vi "ConvertVSEnumToPath.vi"(10 "Source.Path Type":T1(ring), 11 "Path In":path) -> (3 "appended path":path)   [LabVIEW 2015, in "Configuration Tool.lvlib"]
uses:
  Configuration Tool.lvlib
  <vilib>/Utility/sysdir.llb/System Directory Type.ctl
  Global Settings.vi
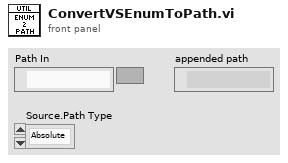
[diagram p1: front panel]
types:
  T1 = enum16{"Absolute", "To Base", "To Common Doc Dir", "To Application Data Dir"}
  T2 = typedef "System Directory Type.ctl" = i32
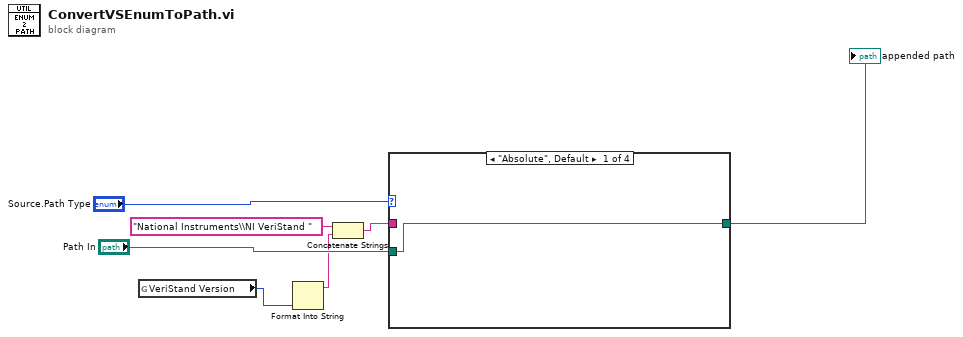
[diagram p0: block diagram]
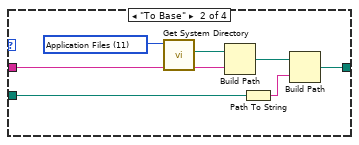
[diagram p2: hidden frame]
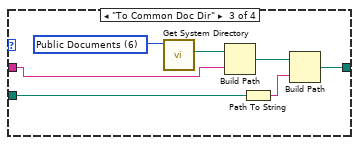
[diagram p3: hidden frame]
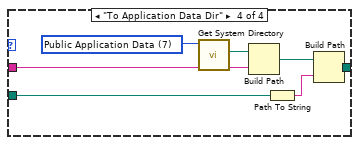
[diagram p4: hidden frame]
diagram:
  n1 = global read "Global Settings.vi" "VeriStand Version"() -> (w4:enum16{"2013", "2014", "2015", "2016"})
  n2 = Format Into String(w4) -> (resulting string=w2:string)  [unwired: 3 in, 1 out]
  n3 = Concatenate Strings("National Instruments\\NI VeriStand " ("name or relative path"), w2) -> (w1:string)
  n4 = case shown="\"Absolute\", Default" "Source.Path Type" {
    tunnel: "Path In" -> [w8 w11 w18 w25]
    tunnel: [w8 w10 w17 w24] -> w7
    tunnel: w1 -> [_ w9 w16 w23]
    frame "Absolute", Default {
    }
    frame "To Base" {
      w15 = T2 11 items=["User Home"=0, "User Desktop"=1, "User Documents"=2, "User Application Data"=3, "User Preferences"=4, "User Temporary"=5, "Public Documents"=6, "Public Application Data"=7, "Public Preferences"=8, "Public Cache"=13, "System Core Libraries"=9, "System Installed Libraries"=10, "Application Files"=11, "Boot Volume Root"=12] ("system directory type")
      n5 = call <vilib>:"Get System Directory.vi"("system directory type"=w15) -> ("system directory"=w14:path)  [unwired: 10 in]
      n6 = Build Path(base path=w14, name or relative path=w9) -> (appended path=w13:path)
      n7 = Path To String(path=w11) -> (string=w12:string)
      n8 = Build Path(base path=w13, name or relative path=w12) -> (appended path=w10:path)
    }
    frame "To Common Doc Dir" {
      w22 = T2 6 items=["User Home"=0, "User Desktop"=1, "User Documents"=2, "User Application Data"=3, "User Preferences"=4, "User Temporary"=5, "Public Documents"=6, "Public Application Data"=7, "Public Preferences"=8, "Public Cache"=13, "System Core Libraries"=9, "System Installed Libraries"=10, "Application Files"=11, "Boot Volume Root"=12] ("system directory type")
      n9 = call <vilib>:"Get System Directory.vi"("system directory type"=w22) -> ("system directory"=w21:path)  [unwired: 10 in]
      n10 = Build Path(base path=w21, name or relative path=w16) -> (appended path=w20:path)
      n11 = Path To String(path=w18) -> (string=w19:string)
      n12 = Build Path(base path=w20, name or relative path=w19) -> (appended path=w17:path)
    }
    frame "To Application Data Dir" {
      w29 = T2 7 items=["User Home"=0, "User Desktop"=1, "User Documents"=2, "User Application Data"=3, "User Preferences"=4, "User Temporary"=5, "Public Documents"=6, "Public Application Data"=7, "Public Preferences"=8, "Public Cache"=13, "System Core Libraries"=9, "System Installed Libraries"=10, "Application Files"=11, "Boot Volume Root"=12] ("system directory type")
      n13 = call <vilib>:"Get System Directory.vi"("system directory type"=w29) -> ("system directory"=w28:path)  [unwired: 10 in]
      n14 = Build Path(base path=w28, name or relative path=w23) -> (appended path=w27:path)
      n15 = Path To String(path=w25) -> (string=w26:string)
      n16 = Build Path(base path=w27, name or relative path=w26) -> (appended path=w24:path)
    }
  }
  "appended path" <- w7
